vi "generate_DAC_voltages_V2.vi"(7 "focus mode?":bool, 8 "derived values":T1, 9 "scan specification":T4={"x amplitude"=0, "x resolution (pixels)"=0, "x offset fly-forward (iterations)"=0, "x offset fly-back (iterations)"=0, "y resolution (nr. of lines)"=0, "y step size"=0, "iterations per pixel"=0, "number of frames"=0, "y offset (pixels)"=0, "number of y-brake lines  (before y-fly-back)"=0, "number y-brake lines (after y-fly-back)"=0, "number of y-fly-back steps"=8, "lines per z step"=0, "number of z/intensity tuples"=0, "number of repetitions (volumes or planes)"=0, "z step size derived"=0, "choose the beginning of z scan"=FALSE, "number of frames (settings)"=0, "FPGA trajectory?"=FALSE}, 10 "counter cluster in":T2, 11 "resonant trigger":bool) -> (0 "acquire?":bool, 1 "fly-back acquisition phase?":bool, 2 "counter cluster out":T2, 3 "DAC voltages":T3 {"ch6" max=4095 step=1; "ch5" max=4095 step=1; "ch4" max=4095 step=1; "ch3" max=4095 step=1; "ch2" max=4095 step=1; "ch1" max=4095 step=1; "ch0" max=4095 step=1})   [LabVIEW 2010]
uses:
  scan_specification_cluster.ctl
  common_typedefs/DAC_voltage_cluster.ctl
  counter_cluster.ctl
  derived_values_cluster.ctl
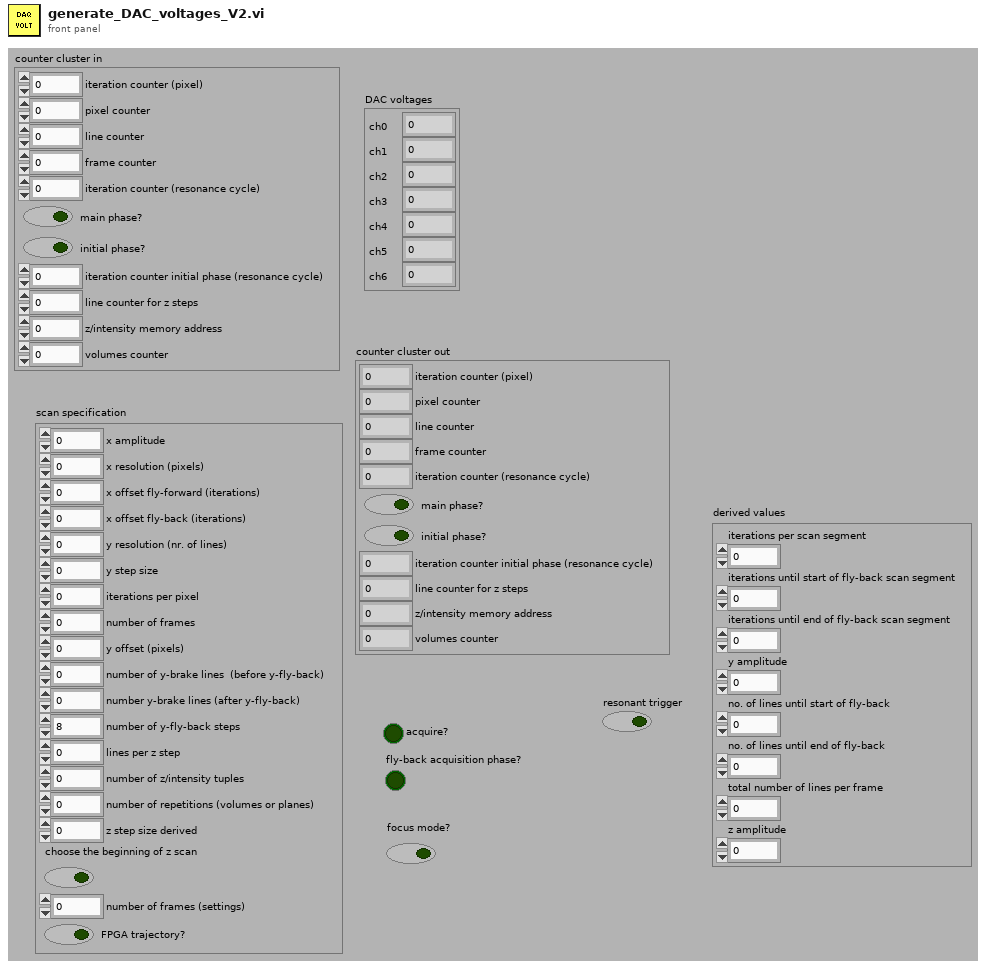
[diagram p1: front panel]
types:
  T1 = typedef "derived_values_cluster.ctl" = cluster{"iterations per scan segment":u16, "iterations until start of fly-back scan segment":u16, "iterations until end of fly-back scan segment":u16, "y amplitude":u16, "no. of lines until start of fly-back":u16, "no. of lines until end of fly-back":u16, "total number of lines per frame ":u16, "z amplitude":u16}
  T2 = typedef "counter_cluster.ctl" = cluster{"iteration counter (pixel)":u16, "pixel counter":u16, "line counter":u16, "frame counter":u16, "iteration counter (resonance cycle)":u16, "main phase?":bool, "initial phase?":bool, "iteration counter initial phase (resonance cycle)":u16, "line counter for z steps":u16, "z/intensity memory address":u32, "volumes counter":u16}
  T3 = typedef "DAC_voltage_cluster.ctl" = cluster{"ch0":u16, "ch1":i16, "ch2":i16, "ch3":u16, "ch4":u16, "ch5":u16, "ch6":u16}
  T4 = typedef "scan_specification_cluster.ctl" = cluster{"x amplitude":u16, "x resolution (pixels)":u16, "x offset fly-forward (iterations)":u16, "x offset fly-back (iterations)":u16, "y resolution (nr. of lines)":u16, "y step size":u16, "iterations per pixel":u16, "number of frames":i32, "y offset (pixels)":u16, "number of y-brake lines  (before y-fly-back)":u16, "number y-brake lines (after y-fly-back)":u16, "number of y-fly-back steps":u16, "lines per z step":u16, "number of z/intensity tuples":u16, "number of repetitions (volumes or planes)":i32, "z step size derived":u16, "choose the beginning of z scan":bool, "number of frames (settings)":i32, "FPGA trajectory?":bool}
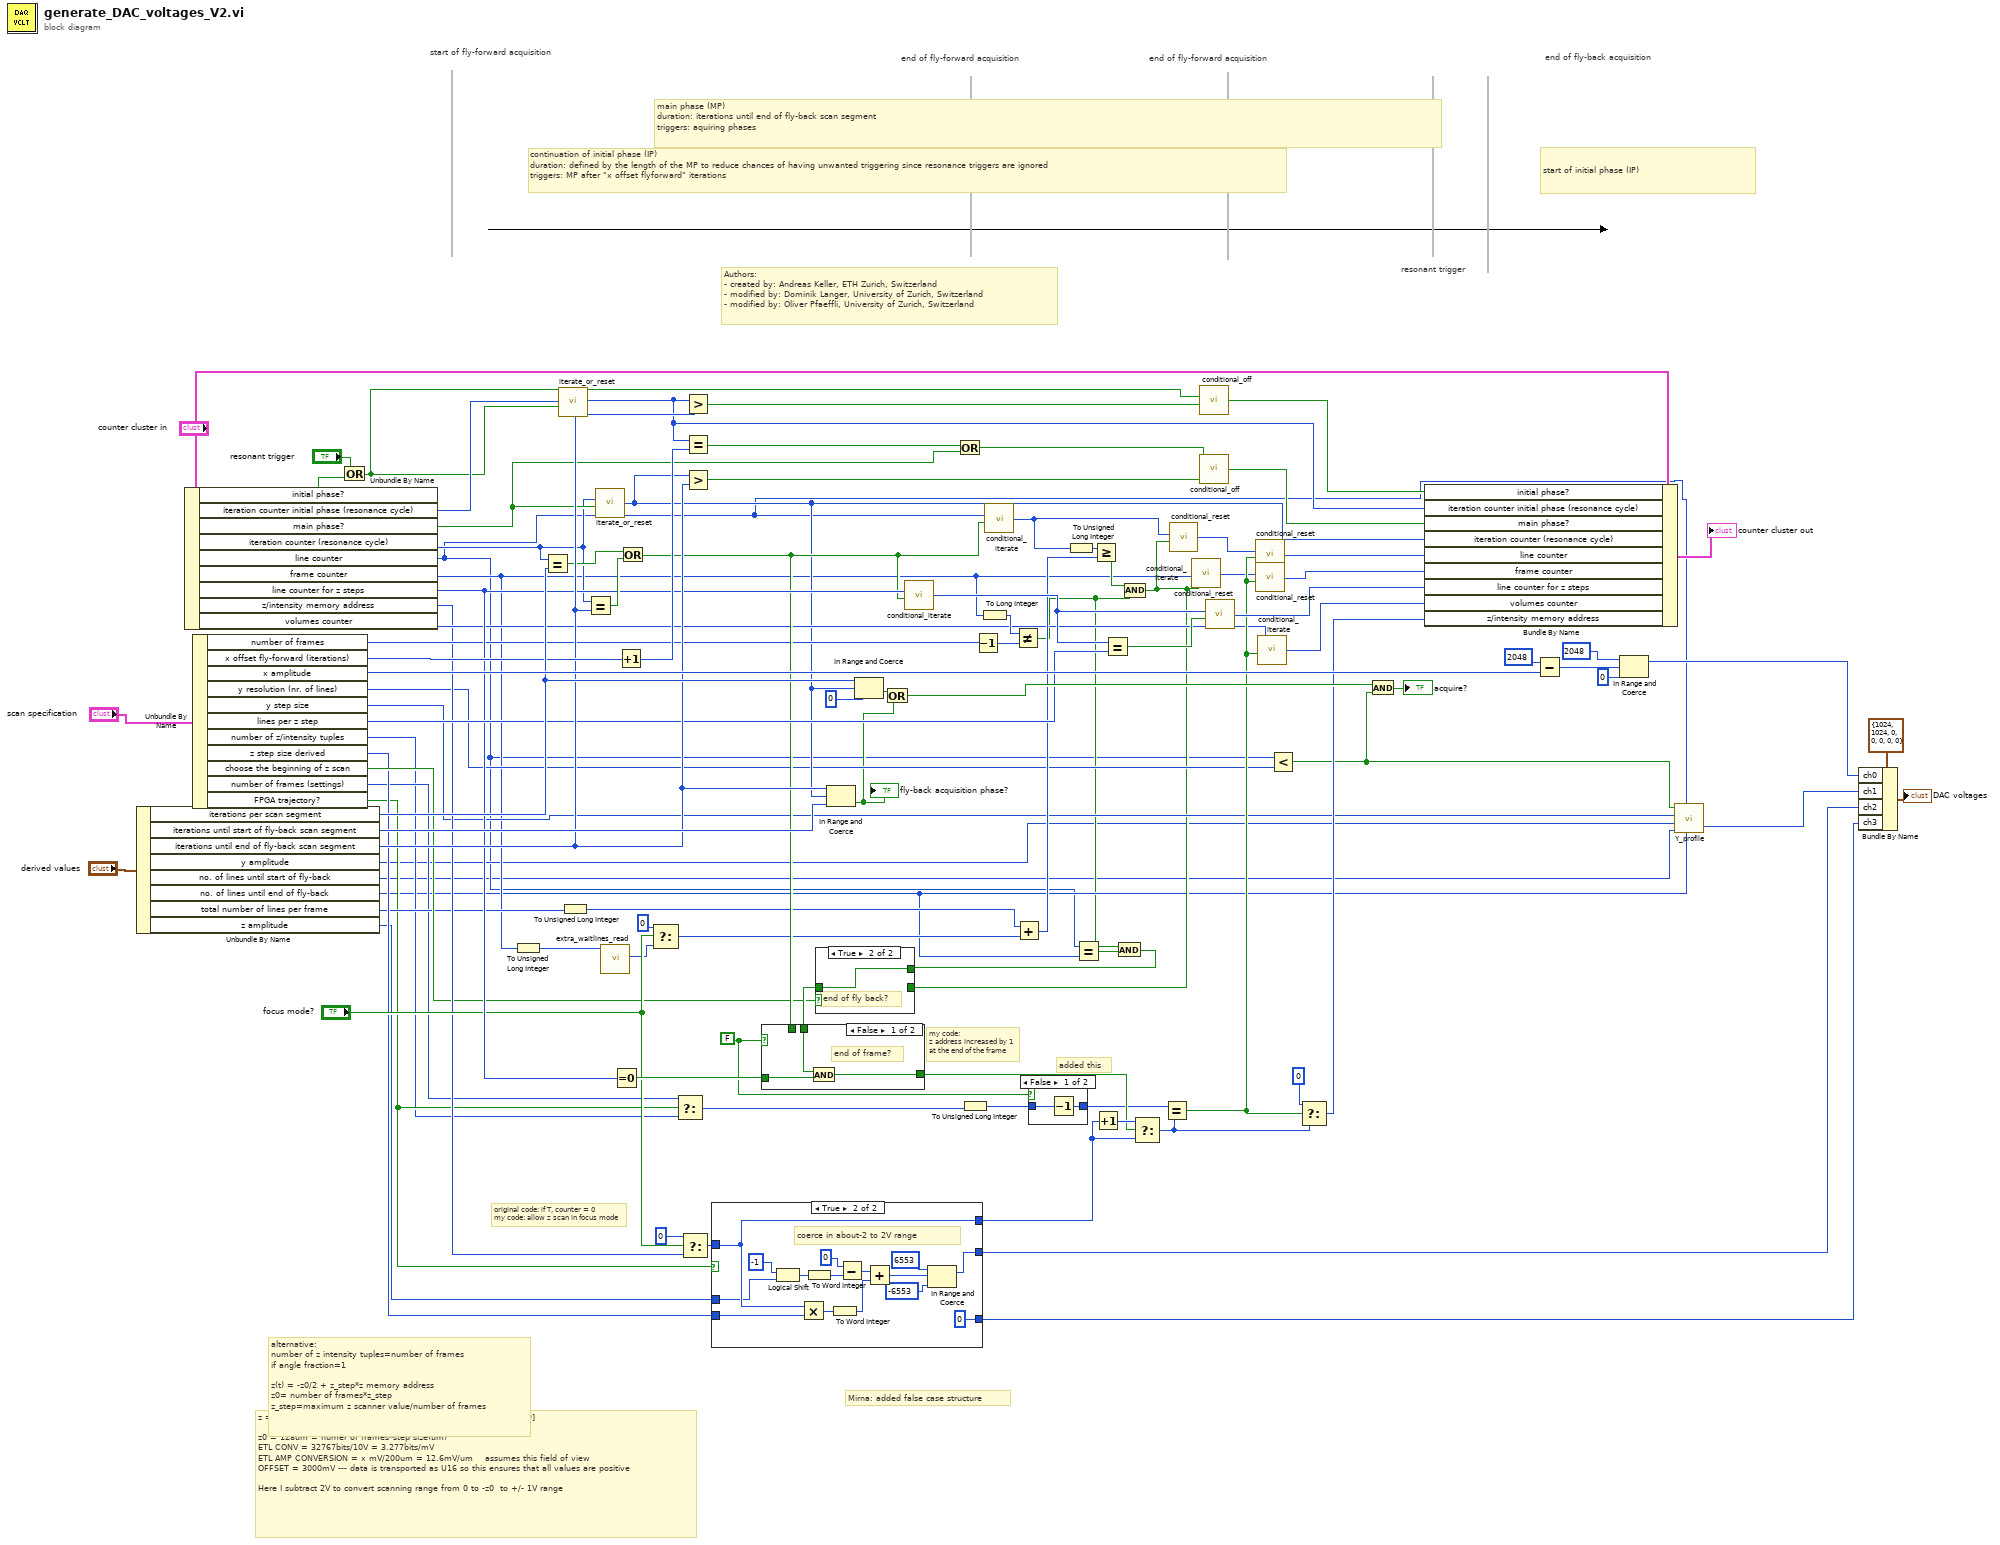
[diagram p0: block diagram]
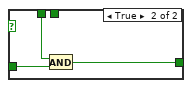
[diagram p4: hidden frame]
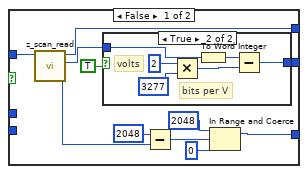
[diagram p5: hidden frame]
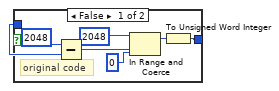
[diagram p6: hidden frame]
diagram:
  w6 = FALSE
  # "added this"
  # "z = ETL CONV [OFFSET - ETL AMPLITUDE CONVERSION*Z0/2(1-COS)]\n\nz0 = 128um = numer of frames*step size(um)\nETL CONV = 32767bits/10V = 3.277bits/mV\nETL AMP CONVERSION = x mV/200um = 12.6mV/um    assumes this field of view\nOFFSET = 3000mV --- data is transported as U16 so this ensures that all values are positive\n\nHere I subtract 2V to convert scanning range from 0 to -z0  to +/- 1V range"
  # "my code:\nz address increased by 1\nat the end of the frame"
  # "alternative:\nnumber of z intensity tuples=number of frames\nif angle fraction=1\n\nz(t) = -z0/2 + z_step*z memory address\nz0= number of frames*z_step\nz_step=maximum z scanner value/number of frames"
  # "original code: if T, counter = 0\nmy code: allow z scan in focus mode"
  # "Mirna: added false case structure"
  # "start of initial phase (IP)"
  # "continuation of initial phase (IP)\nduration: defined by the length of the MP to reduce chances of having unwanted triggering since resonance triggers are ignored\ntriggers: MP after \"x offset flyforward\" iterations"
  # "end of fly-back acquisition"
  # "end of fly-forward acquisition"
  # "end of fly-forward acquisition"
  # "start of fly-forward acquisition"
  # "main phase (MP)\nduration: iterations until end of fly-back scan segment\ntriggers: aquiring phases"
  # "resonant trigger"
  # "Authors: \n- created by: Andreas Keller, ETH Zurich, Switzerland\n- modified by: Dominik Langer, University of Zurich, Switzerland\n- modified by: Oliver Pfaeffli, University of Zurich, Switzerland"
  n1 = Unbundle By Name("derived values") -> ("iterations per scan segment"=w83:u16, "iterations until start of fly-back scan segment"=w86:u16, "iterations until end of fly-back scan segment"=w72:u16, "y amplitude"=w3:u16, "no. of lines until start of fly-back"=w1:u16, "no. of lines until end of fly-back"=w11:u16, "total number of lines per frame"=w24:u16, "z amplitude"=w4:u16)
  n2 = Unbundle By Name("counter cluster in") -> ("initial phase?"=w85:bool, "iteration counter initial phase (resonance cycle)"=w81:u16, "main phase?"=w41:bool, "iteration counter (resonance cycle)"=w32:u16, "line counter"=w2:u16, "frame counter"=w23:u16, "line counter for z steps"=w65:u16, "z/intensity memory address"=w35:u32, "volumes counter"=w44:u16)
  n3 = Unbundle By Name("scan specification") -> ("number of frames"=w51:i32, "x offset fly-forward (iterations)"=w75:u16, "x amplitude"=w89:u16, "y resolution (nr. of lines)"=w33:u16, "y step size"=w29:u16, "lines per z step"=w69:u16, "number of z/intensity tuples"=w13:u16, "z step size derived"=w25:u16, "choose the beginning of z scan"=w26:bool, "number of frames (settings)"=w14:i32, "FPGA trajectory?"=w15:bool)
  n4 = Or(x="resonant trigger", y=w85) -> (x .or. y?=w79:bool)
  n5 = To Unsigned Long Integer(number=w23) -> (unsigned 32bit integer=w57:u32)
  n6 = Equal?(x=w32, y=w83) -> (x = y?=w70:bool)
  n7 = call "iterate_or_reset.vi"("iterate?"=w79, "number in"=w81) -> ("number out"=w20:u16)  [unwired: 4 in]
  n8 = To Unsigned Long Integer(number=w24) -> (unsigned 32bit integer=w21:u32)
  n9 = Equal?(x=w32, y=w72) -> (x = y?=w71:bool)
  n10 = call "iterate_or_reset.vi"("iterate?"=w41, "number in"=w32) -> ("number out"=w40:u16)  [unwired: 4 in]
  n11 = call "extra_waitlines_read.vi"("address extra waitlines IN"=w57) -> ("extra waitline data"=w8:u32)  [unwired: 9 in, 1 out]
  n12 = Equal To 0?(x=w65) -> (x = 0?=w60:bool)
  n13 = Increment(x=w75) -> (x+1=w74:u16)
  n14 = Or(x=w70, y=w71) -> (x .or. y?=w59:bool)
  n15 = Select(t=u32 0, s="focus mode?", f=w8) -> (s? t:f=w46:u32)
  n16 = Select(t=w14, s=w15, f=w13) -> (s? t:f=w34:i32)
  n17 = Select(t=u32 0, s="focus mode?", f=w35) -> (s? t:f=w36:u32)
  n18 = Greater?(x=w20, y=w72) -> (0:w73:bool)
  n19 = Equal?(x=w20, y=w74) -> (x = y?=w80:bool)
  n20 = Greater?(x=w40, y=w72) -> (0:w77:bool)
  n21 = case shown="True" w15 {
    tunnel: [w106 u16 0 ("intensity")] -> w38
    tunnel: [w112 w138] -> w58
    tunnel: [w103 w130] -> w37
    tunnel: w36 -> [w111 w138]
    tunnel: w25 -> [_ w139]
    tunnel: w4 -> [_ w127]
    frame False {
      n22 = call "z_scan_read.vi"("address in"=w111) -> ("intensity"=w109:u16, "z-value"=w104:i16, "address out"=w112:u32)  [unwired: 8 in]
      n23 = case shown="True" TRUE {
        tunnel: w104 -> [w113 w125]
        tunnel: [w114 w124] -> w103
        frame False {
          # "original code"
          n24 = Subtract(x=i16 2048, y=w113) -> (x-y=w115:i16)
          n25 = In Range and Coerce(upper limit=i16 2048, x=w115, lower limit=i16 0) -> (coerced(x)=w116:i16)  [unwired: 1 out]
          n26 = To Unsigned Word Integer(number=w116) -> (unsigned 16bit integer=w114:u16)
        }
        frame True {
          # "bits per V"
          # "volts"
          n27 = Multiply(x=i16 2 ("y"), y=i16 3277) -> (x*y=w122:i16)
          n28 = To Word Integer(number=w125) -> (16bit integer=w120:i16)
          n29 = Subtract(x=w120, y=w122) -> (x-y=w124:i16)
        }
      }
      n30 = Subtract(x=i16 2048, y=w109) -> (x-y=w105:u16)
      n31 = In Range and Coerce(upper limit=u16 2048, x=w105, lower limit=u16 0) -> (coerced(x)=w106:u16)  [unwired: 1 out]
    }
    frame True {
      # "coerce in about-2 to 2V range"
      n32 = Logical Shift(y=i16 -1 ("n"), x=w127) -> (x << y=w128:u16)
      n33 = Multiply(x=w138, y=w139) -> (x*y=w136:u32)
      n34 = To Word Integer(number=w128) -> (16bit integer=w135:i16)
      n35 = To Word Integer(number=w136) -> (16bit integer=w134:i16)
      n36 = Subtract(x=i16 0, y=w135) -> (x-y=w137:i16)
      n37 = Add(x=w137, y=w134) -> (x+y=w131:i16)
      n38 = In Range and Coerce(upper limit=i16 6553, x=w131, lower limit=i16 -6553) -> (coerced(x)=w130:i16)  [unwired: 1 out]
    }
  }
  n39 = In Range and Coerce(upper limit=w72, x=w40, lower limit=w86) -> (In Range?=w18:bool)  [unwired: 1 out]
  "fly-back acquisition phase?" <- w18
  n40 = In Range and Coerce(upper limit=w83, x=w40, lower limit=u16 0) -> (In Range?=w97:bool)  [unwired: 1 out]
  n41 = Or(x=w97, y=w18) -> (x .or. y?=w88:bool)
  n42 = call "conditional_iterate.vi"("iterate?"=w59, "number in"=w65) -> ("number out"=w66:u16)  [unwired: 4 in]
  n43 = Or(x=w80, y=w41) -> (x .or. y?=w42:bool)
  n44 = To Unsigned Long Integer(number=w34) -> (unsigned 32bit integer=w63:u32)
  n45 = Decrement(x=w51) -> (x-1=w50:i32)
  n46 = To Long Integer(number=w23) -> (32bit integer=w49:i32)
  n47 = call "conditional_iterate.vi"("iterate?"=w59, "number in"=w2) -> ("number out"=w10:u16)  [unwired: 4 in]
  n48 = Not Equal?(x=w49, y=w50) -> (x != y?=w9:bool)
  n49 = Add(x=w21, y=w46) -> (x+y=w47:u32)
  n50 = case shown="False" w6 {
    tunnel: w63 -> [w142 w143]
    tunnel: [w141 w143] -> w7
    frame False {
      n51 = Decrement(x=w142) -> (x-1=w141:u32)
    }
    frame True {
    }
  }
  n52 = To Unsigned Long Integer(number=w10) -> (unsigned 32bit integer=w12:u32)
  n53 = Equal?(x=w2, y=w11) -> (x = y?=w16:bool)
  n54 = Greater Or Equal?(x=w12, y=w47) -> (x >= y?=w52:bool)
  n55 = Increment(x=w58) -> (x+1=w64:u32)
  n56 = Equal?(x=w66, y=w69) -> (x = y?=w67:bool)
  n57 = And(x=w9, y=w16) -> (x .and. y?=w17:bool)
  n58 = And(x=w52, y=w9) -> (x .and. y?=w28:bool)
  n59 = case shown="True" w26 {
    tunnel: w17 -> [_ w145]
    tunnel: w28 -> [w144 _]
    tunnel: [w144 w145] -> w27
    frame False {
      # "end of frame?"
    }
    frame True {
      # "end of fly back?"
    }
  }
  n60 = case shown="False" w6 {
    tunnel: w60 -> [w148 w151]
    tunnel: w59 -> [_ w150]
    tunnel: [w147 w149] -> w22
    tunnel: w27 -> [w146 _]
    frame False {
      # "end of frame?"
      n61 = And(x=w146, y=w148) -> (x .and. y?=w147:bool)
    }
    frame True {
      n62 = And(x=w150, y=w151) -> (x .and. y?=w149:bool)
    }
  }
  n63 = Select(t=w64, s=w22, f=w58) -> (s? t:f=w62:u32)
  n64 = Equal?(x=w7, y=w62) -> (x = y?=w48:bool)
  n65 = call "conditional_reset.vi"("reset?"=w28, "number in"=w10) -> ("number out"=w54:u16)  [unwired: 4 in]
  n66 = call "conditional_iterate.vi"("iterate?"=w28, "number in"=w23) -> ("number out"=w30:u16)  [unwired: 4 in]
  n67 = call "conditional_off.vi"("switch off?"=w73, "boolean in"=w79) -> ("boolean out"=w78:bool)  [unwired: 4 in]
  n68 = call "conditional_off.vi"("switch off?"=w77, "boolean in"=w42) -> ("boolean out"=w76:bool)  [unwired: 4 in]
  n69 = call "conditional_reset.vi"("reset?"=w67, "number in"=w66) -> ("number out"=w68:u16)  [unwired: 4 in]
  n70 = call "conditional_reset.vi"("reset?"=w48, "number in"=w54) -> ("number out"=w53:u16)  [unwired: 4 in]
  n71 = call "conditional_reset.vi"("reset?"=w48, "number in"=w30) -> ("number out"=w31:u16)  [unwired: 4 in]
  n72 = call "conditional_iterate.vi"("iterate?"=w48, "number in"=w44) -> ("number out"=w55:u16)  [unwired: 4 in]
  n73 = Less?(x=w2, y=w33) -> (x < y?=w19:bool)
  n74 = Select(t=u32 0, s=w48, f=w62) -> (s? t:f=w56:u32)
  n75 = And(x=w88, y=w19) -> (x .and. y?=→"acquire?":bool)
  n76 = Bundle By Name(cluster="counter cluster in", "initial phase?"=w78, "iteration counter initial phase (resonance cycle)"=w20, "main phase?"=w76, "iteration counter (resonance cycle)"=w40, "line counter"=w53, "frame counter"=w31, "line counter for z steps"=w68, "volumes counter"=w55, "z/intensity memory address"=w56) -> (→"counter cluster out":T2)
  n77 = Subtract(x=u16 2048, y=w89) -> (x-y=w93:u16)
  n78 = In Range and Coerce(upper limit=u16 2048, x=w93, lower limit=u16 0) -> (coerced(x)=w92:u16)  [unwired: 1 out]
  n79 = call "Y_profile.vi"("no. of lines until end of fly-back"=w11, "line counter"=w2, "no. of lines until start of fly-back"=w1, "y amplitude"=w3, "y step size"=w29, "true when line counter smaller than y resolution"=w19) -> ("y signal"=w39:i16)  [unwired: 1 in]
  n80 = Bundle By Name(cluster=T3 {"ch0"=1024, "ch1"=1024, "ch2"=0, "ch3"=0, "ch4"=0, "ch5"=0, "ch6"=0} ("DAC voltage"), "ch0"=w92, "ch1"=w39, "ch2"=w37, "ch3"=w38) -> (→"DAC voltages":T3)
